vi "Common-SecondToCountDownString.vi"(4 "秒":u32) -> (1 "倒计时字符串":string)   [LabVIEW 2014]
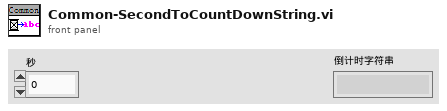
[diagram p1: front panel]
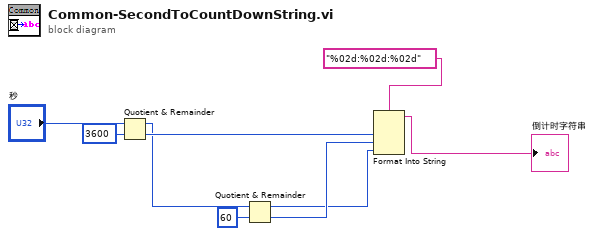
[diagram p0: block diagram]
diagram:
  n1 = Quotient & Remainder(x="秒", y=u32 3600) -> (x-y*floor(x/y)=w1:u32, floor(x/y)=w5:u32)
  n2 = Quotient & Remainder(x=w1, y=u32 60) -> (x-y*floor(x/y)=w3:u32, floor(x/y)=w4:u32)
  n3 = Format Into String(format string="%02d:%02d:%02d" ("格式字符串"), w5, w4, w3) -> (resulting string=→"倒计时字符串":string)  [unwired: 2 in, 1 out]
